vi "PXI-StopDAQ.vi"(4 "error in (no error)":errorcluster, 5 "Reset (T)":bool=TRUE, 7 "Wait for DAQ to stop? (T)":bool=TRUE) -> (0 "error out":errorcluster)   [LabVIEW 2020]
doc: "Sets global variables that terminate the main DAQ loop."
uses:
  DAQ Engine VIs/PXI Globals.vi
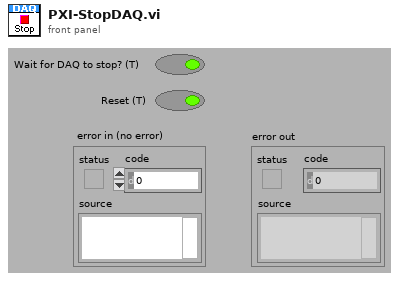
[diagram p1: front panel]
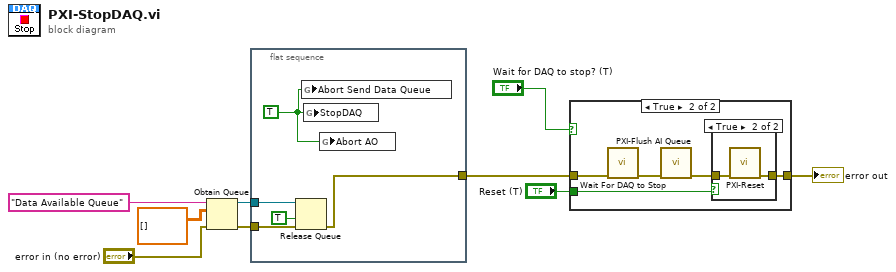
[diagram p0: block diagram]
diagram:
  n1 = Obtain Queue(name (unnamed)="Data Available Queue", element data type=dbl[][] [] ("AI Waveforms 2"), error in (no error)="error in (no error)") -> (queue out=w4:refnum<queue>, error out=w3:errorcluster)  [unwired: 2 in, 1 out]
  n2 = flat-sequence {
    tunnel: [w11] -> w9
    tunnel: w4 -> [w14]
    tunnel: w3 -> [w13]
    frame #0 {
      w10 = TRUE ("StopDAQ")
      n3 = Release Queue(queue=w14, force destroy? (F)=TRUE, error in (no error)=w13) -> (error out=w11:errorcluster)  [unwired: 2 out]
      n4 = global write "PXI Globals.vi" "Abort Send Data Queue"(w10) -> ()
      n5 = global write "PXI Globals.vi" "StopDAQ"(w10) -> ()
      n6 = global write "PXI Globals.vi" "Abort AO"(w10) -> ()
    }
  }
  n7 = case shown="True" "Wait for DAQ to stop? (T)" {
    tunnel: w9 -> [w15 w20]
    tunnel: [w15 w17] -> w2
    tunnel: "Reset (T)" -> [_ w16]
    frame False {
    }
    frame True {
      n8 = call "Wait For DAQ to Stop.vi"("error in (no error)"=w20) -> ("error out"=w19:errorcluster)  [unwired: 10 in]
      n9 = call "PXI-Flush AI Queue.vi"("error in (no error)"=w19) -> ("error out"=w18:errorcluster)  [unwired: 14 in]
      n10 = case shown="True" w16 {
        tunnel: w18 -> [w21 w23]
        tunnel: [w21 w22] -> w17
        frame False {
        }
        frame True {
          n11 = call "PXI-Reset.vi"("error in (no error)"=w23) -> ("error out"=w22:errorcluster)  [unwired: 10 in]
        }
      }
    }
  }
  "error out" <- w2
